vi "Create Chunk ASCII or Unicode.vi"(0 "Character type":T1=enum."ASCII", 7 "Text":string, 11 "error in (no error)":errorcluster) -> (8 "Phrase refnum":refnum<k24>, 10 "Char U16 [ ]":u16[](array[numeric]) format="%04x", 15 "error out":errorcluster)   [LabVIEW 2019]
doc: "Developed by Jean-Marc Simard\nCopyright © 2012, Exaprom Inc.\nAll rights reserved.\nLicense: BSD\n\nWith iTextSharp 4.1.6 (http://itextsharp.sourceforge.net)\nunder Mozilla Public License Version 1.1\n(http://www.mozilla.org/MPL/MPL-1.1.html)"
uses:
  C:/Program Files/National Instruments/LabVIEW 2019/user.lib/Exaprom PDF/DLL/itextsharp.dll
  DLL/itextsharp.dll
  <userlib>/Exaprom PDF/Controls/Text Controls/Unicode/Type and run direction.ctl
panel:
  in  "Char U16 [ ] 2":u16[](array[numeric]) format="%04x"
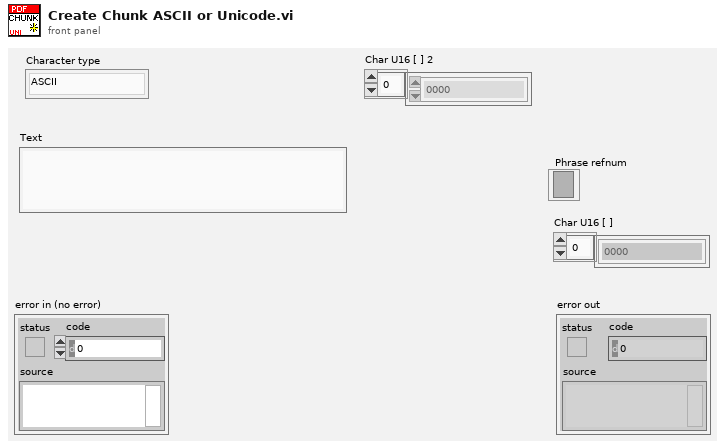
[diagram p1: front panel]
types:
  T1 = typedef "Type and run direction.ctl" = enum16{"Select", "ASCII", "UTF-16", "UTF-16 (default)", "UTF-16 (LTR)", "UTF-16 (RTL)"}
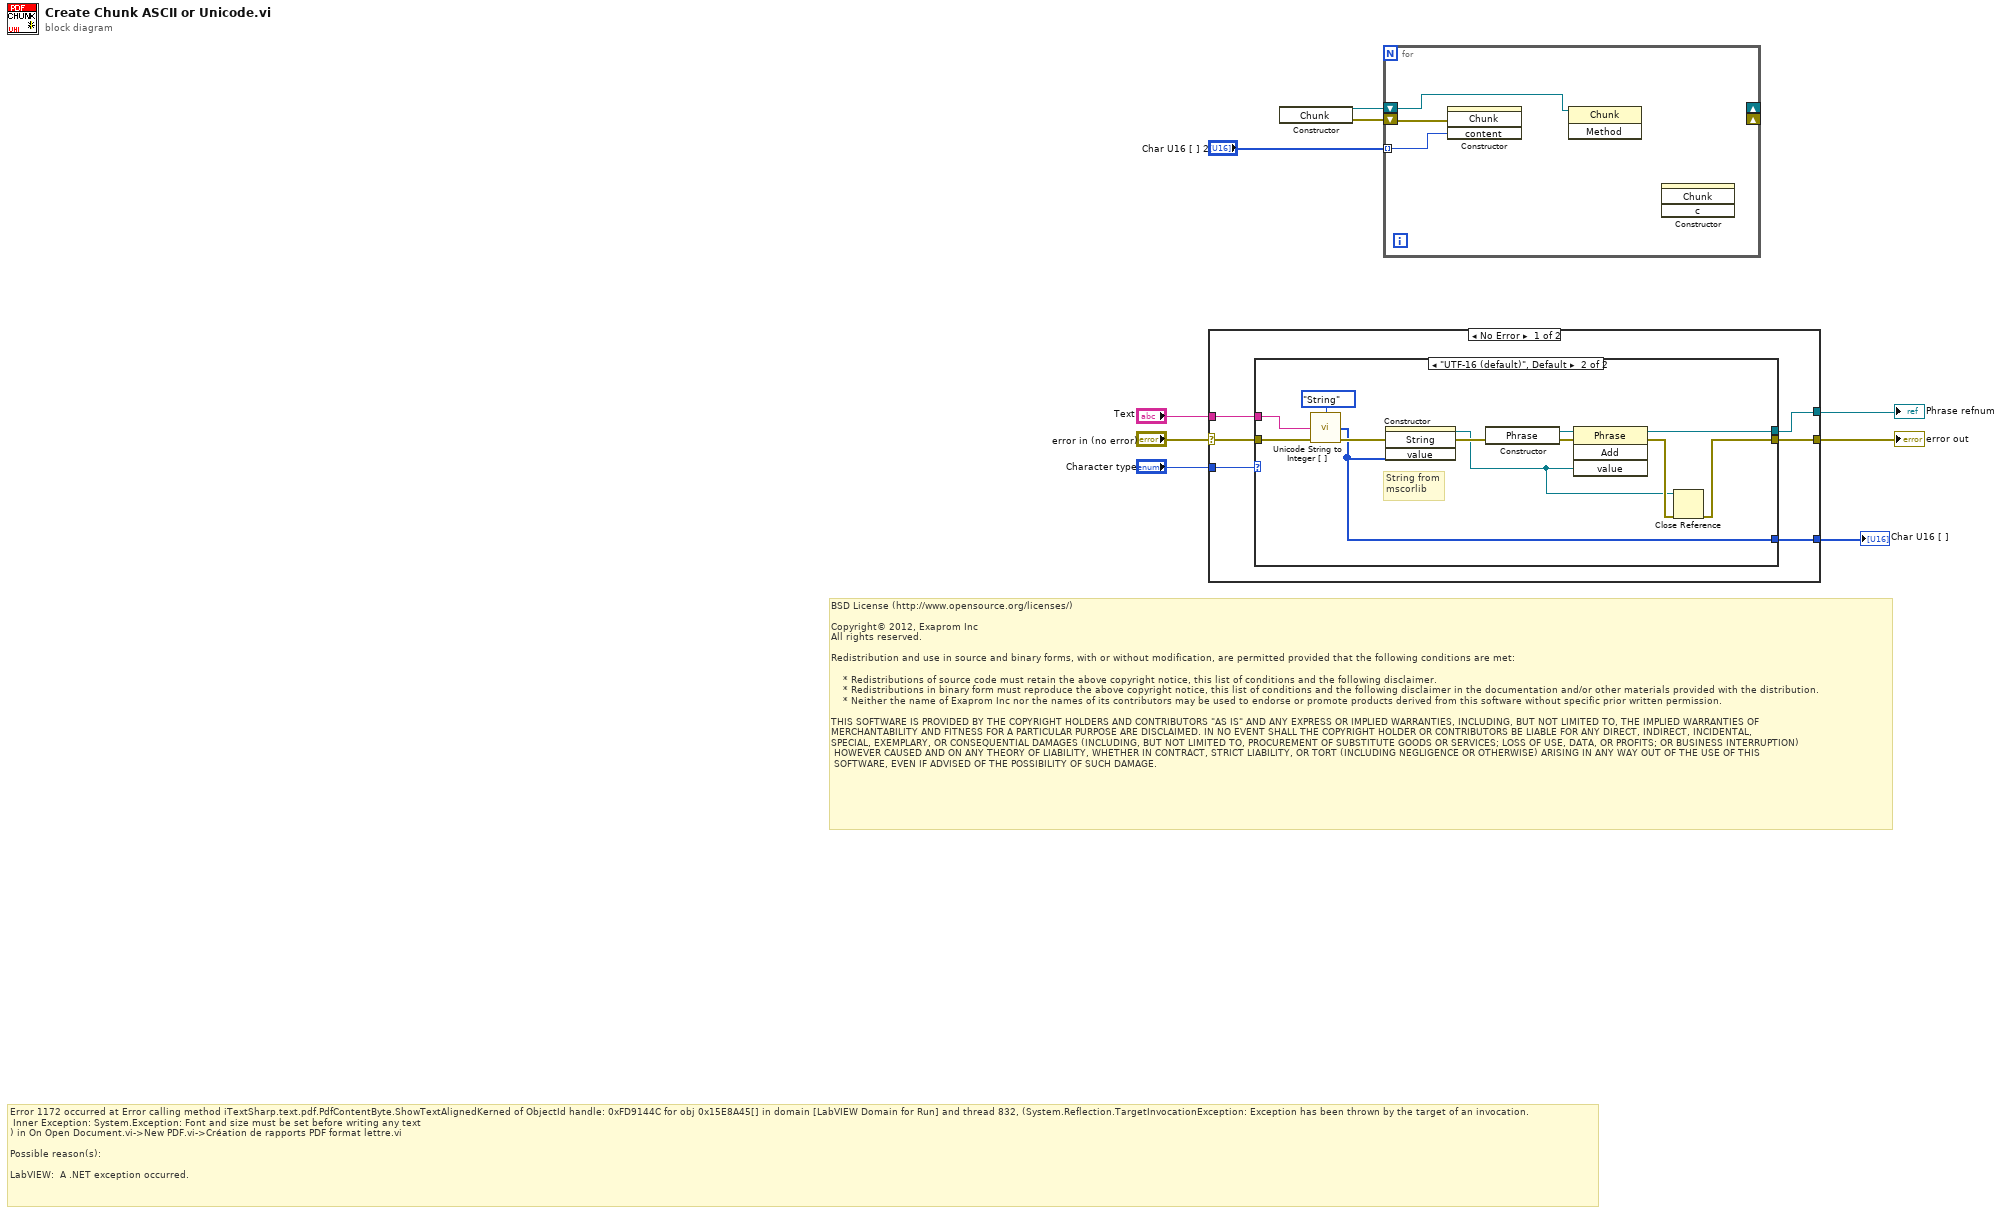
[diagram p0: block diagram]
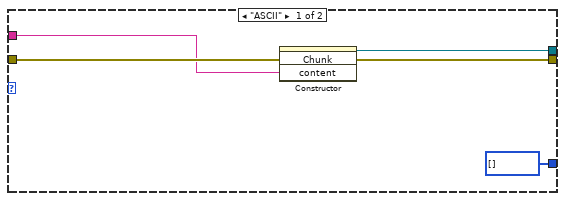
[diagram p2: hidden frame]
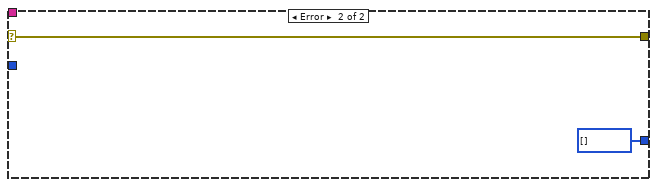
[diagram p3: hidden frame]
diagram:
  # "Error 1172 occurred at Error calling method iTextSharp.text.pdf.PdfContentByte.ShowTextAlignedKerned of ObjectId handle: 0xFD9144C for obj 0x15E8A45[] in domain [LabVIEW Domain for Run] and thread 832, (System.Reflection.TargetInvocationException: Exception has been thrown by the target of an invocation.\n\tInner Exception: System.Exception: Font and size must be set before writing any text\n) in On Open Document.vi->New PDF.vi->Création de rapports PDF format lettre.vi\n\nPossible reason(s):\n\nLabVIEW:  A .NET exception occurred."
  # "BSD License (http://www.opensource.org/licenses/)\n\nCopyright© 2012, Exaprom Inc\nAll rights reserved.\n\nRedistribution and use in source and binary forms, with or without modification, are permitted provided that the following conditions are met:\n\n    * Redistributions of source code must retain the above copyright notice, this list of conditions and the following disclaimer.\n    * Redistributions in binary form must reproduce the above copyright notice, this list of conditions and the following disclaimer in the documentation and/or other materials provided with the distribution.\n    * Neither the name of Exaprom Inc nor the names of its contributors may be used to endorse or promote products derived from this software without specific prior written permission.\n\nTHIS SOFTWARE IS PROVIDED BY THE COPYRIGHT HOLDERS AND CONTRIBUTORS \"AS IS\" AND ANY EXPRESS OR IMPLIED WARRANTIES, INCLUDING, BUT NOT LIMITED TO, THE IMPLIED WARRANTIES OF \nMERCHANTABILITY AND FITNESS FOR A PARTICULAR PURPOSE ARE DISCLAIMED. IN NO EVENT SHALL THE COPYRIGHT HOLDER OR CONTRIBUTORS BE LIABLE FOR ANY DIRECT, INDIRECT, INCIDENTAL,\nSPECIAL, EXEMPLARY, OR CONSEQUENTIAL DAMAGES (INCLUDING, BUT NOT LIMITED TO, PROCUREMENT OF SUBSTITUTE GOODS OR SERVICES; LOSS OF USE, DATA, OR PROFITS; OR BUSINESS INTERRUPTION)\n HOWEVER CAUSED AND ON ANY THEORY OF LIABILITY, WHETHER IN CONTRACT, STRICT LIABILITY, OR TORT (INCLUDING NEGLIGENCE OR OTHERWISE) ARISING IN ANY WAY OUT OF THE USE OF THIS\n SOFTWARE, EVEN IF ADVISED OF THE POSSIBILITY OF SUCH DAMAGE."
  n1 = case shown="No Error" "error in (no error)" {
    selector: "error in (no error)" -> [w13 w34]
    tunnel: [w14 w34] -> w9
    tunnel: "Character type" -> [w15 _]
    tunnel: [w12 _] -> w6
    tunnel: "Text" -> [w11 _]
    tunnel: [w10 u16[] [] ("Char U16 [ ]")] -> w4
    frame No Error {
      n2 = case shown="\"UTF-16 (default)\", Default" w15 {
        tunnel: w13 -> [w20 w25]
        tunnel: [w17 w31] -> w12
        tunnel: [w19 w30] -> w14
        tunnel: w11 -> [w16 w23]
        tunnel: [u16[] [] ("Char U16 [ ]") w21] -> w10
        frame "ASCII" {
          n3 = constructor class="Chunk"(error in=w20, "content"=w16) -> (reference out=w17:refnum<k24>, error out=w19:errorcluster)  [unwired: 2 in, 2 out]
        }
        frame "UTF-16 (default)", Default {
          # "String from\nmscorlib"
          n4 = call <userlib>:"Unicode String to Integer [ ].vi"("From"=enum16{"String", "U16 [ ]"}."String", "Unicode String"=w23, "error in (no error)"=w25) -> ("Char U16 [ ]"=w21:u16[], "error duplicate"=w24:errorcluster)  [unwired: 10 in, 1 out]
          n5 = constructor class="String" ("Constructor Node")(error in=w24, "value"=w21) -> (reference out=w28:refnum<k24>, error out=w32:errorcluster)  [unwired: 2 in, 2 out]
          n6 = constructor class="Phrase"(error in=w32) -> (reference out=w27:refnum<k24>, error out=w26:errorcluster)  [unwired: 2 in, 1 out]
          n7 = invoke class="Phrase" method="Add"(reference=w27, error in=w26, "value"=w28) -> (reference out=w31:refnum<k24>, error out=w29:errorcluster)  [unwired: 1 in, 2 out]
          n8 = Close Reference(reference=w28, error in (no error)=w29) -> (error out=w30:errorcluster)
        }
      }
    }
    frame Error {
    }
  }
  "error out" <- w9
  "Phrase refnum" <- w6
  "Char U16 [ ]" <- w4
  n9 = constructor class="Chunk"() -> (reference out=w2:refnum<k24>, error out=w3:errorcluster)  [unwired: 3 in, 1 out]
  n10 = for {
    shift-right: _ -> [_]
    shift-left: w2 -> [w35]
    shift-right: _ -> [_]
    shift-left: w3 -> [w37]
    tunnel: "Char U16 [ ] 2" -> [w36] mode=indexing
    n11 = constructor class="Chunk"(error in=w37, "content"=w36) -> ()  [unwired: 2 in, 4 out]
    n12 = invoke class="Chunk" method=#-1(reference=w35) -> ()  [unwired: 2 in, 3 out]
    n13 = constructor class="Chunk"() -> ()  [unwired: 3 in, 5 out]
  }
